vi "DC Dfficiency_noTorqueInput.vi"(0 "data":waveform(dbl)[](array[waveform])=[{"t0"=timestamp(3695322048.688499 s since 1904-01-01), "dt"=0.01, "Y"=[27.030278258476777, 27.030278258476777, 27.030278258476777, 27.030278258476777, 27.030278258476777, 27.030278258476777], "attributes"=variant("NI_ChannelName"=variant(string "T_comp_in"), "NI_UnitDescription"=variant(string "Deg C"))}, {"t0"=timestamp(3695322048.688499 s since 1904-01-01), "dt"=0.01, "Y"=[101.4755306317151, 101.4755306317151, 101.4755306317151, 101.4755306317151, 101.4755306317151, 101.4755306317151], "attributes"=variant("NI_ChannelName"=variant(string "T_comp_out"), "NI_UnitDescription"=variant(string "Deg C"))}, {"t0"=timestamp(3695322048.688499 s since 1904-01-01), "dt"=0.01, "Y"=[74.8524982036163, 74.8524982036163, 74.8524982036163, 74.8524982036163, 74.8524982036163, 74.8524982036163], "attributes"=variant("NI_ChannelName"=variant(string "T_int"), "NI_UnitDescription"=variant(string "Deg C"))}, {"t0"=timestamp(3695322048.688499 s since 1904-01-01), "dt"=0.01, "Y"=[49.22287356053607, 49.22287356053607, 49.22287356053607, 49.22287356053607, 49.22287356053607, 49.22287356053607], "attributes"=variant("NI_ChannelName"=variant(string "T_vapor"), "NI_UnitDescription"=variant(string "Deg C"))}, {"t0"=timestamp(3695322048.688499 s since 1904-01-01), "dt"=0.01, "Y"=[22.86482944196074, 22.86482944196074, 22.86482944196074, 22.86482944196074, 22.86482944196074, 22.86482944196074], "attributes"=variant("NI_ChannelName"=variant(string "T_cd_out"), "NI_UnitDescription"=variant(string "Deg C"))}, {"t0"=timestamp(3695322048.688499 s since 1904-01-01), "dt"=0.01, "Y"=[22.390101755165144, 22.390101755165144, 22.390101755165144, 22.390101755165144, 22.390101755165144, 22.390101755165144], "attributes"=variant("NI_ChannelName"=variant(string "T_liq"), "NI_UnitDescription"=variant(string "Deg C"))}, {"t0"=timestamp(3695322048.688499 s since 1904-01-01), "dt"=0.01, "Y"=[22.35929456927789, 22.35929456927789, 22.35929456927789, 22.35929456927789, 22.35929456927789, 22.35929456927789], "attributes"=variant("NI_ChannelName"=variant(string "T_cf_in"), "NI_UnitDescription"=variant(string "Deg C"))}, {"t0"=timestamp(3695322048.688499 s since 1904-01-01), "dt"=0.01, "Y"=[25.57925048739495, 25.57925048739495, 25.57925048739495, 25.57925048739495, 25.57925048739495, 25.57925048739495], "attributes"=variant("NI_ChannelName"=variant(string "T_cf_out"), "NI_UnitDescription"=variant(string "Deg C"))}, {"t0"=timestamp(3695322048.688499 s since 1904-01-01), "dt"=0.01, "Y"=[-56050.12537094423, -56050.12537094423, -56050.12537094423, -56050.12537094423, -56050.12537094423, -56050.12537094423], "attributes"=variant("NI_ChannelName"=variant(string "T_cj_in"), "NI_UnitDescription"=variant(string "Deg C"))}, {"t0"=timestamp(3695322048.688499 s since 1904-01-01), "dt"=0.01, "Y"=[-56050.12537094423, -56050.12537094423, -56050.12537094423, -56050.12537094423, -56050.12537094423, -56050.12537094423], "attributes"=variant("NI_ChannelName"=variant(string "T_cj_out"), "NI_UnitDescription"=variant(string "Deg C"))}, {"t0"=timestamp(3695322048.688499 s since 1904-01-01), "dt"=0.01, "Y"=[25.130324713777938, 25.130324713777938, 25.130324713777938, 25.130324713777938, 25.130324713777938, 25.130324713777938], "attributes"=variant("NI_ChannelName"=variant(string "T_amb"), "NI_UnitDescription"=variant(string "Deg C"))}, {"t0"=timestamp(3695322048.688499 s since 1904-01-01), "dt"=0.01, "Y"=[89.88480677591595, 89.88480677591595, 89.88480677591595, 89.88480677591595, 89.88480677591595, 89.88480677591595], "attributes"=variant("NI_ChannelName"=variant(string "T_os_out"), "NI_UnitDescription"=variant(string "Deg C"))}, {"t0"=timestamp(3695322048.688499 s since 1904-01-01), "dt"=0.01, "Y"=[66.71254591399129, 66.71254591399129, 66.71254591399129, 66.71254591399129, 66.71254591399129, 66.71254591399129], "attributes"=variant("NI_ChannelName"=variant(string "Housing Upstream"), "NI_UnitDescription"=variant(string "Deg C"))}, {"t0"=timestamp(3695322048.688499 s since 1904-01-01), "dt"=0.01, "Y"=[76.6589685879223, 76.6589685879223, 76.6589685879223, 76.6589685879223, 76.6589685879223, 76.6589685879223], "attributes"=variant("NI_ChannelName"=variant(string "Housing Middle"), "NI_UnitDescription"=variant(string "Deg C"))}, {"t0"=timestamp(3695322048.688499 s since 1904-01-01), "dt"=0.01, "Y"=[72.22038712366484, 72.22038712366484, 72.22038712366484, 72.22038712366484, 72.22038712366484, 72.22038712366484], "attributes"=variant("NI_ChannelName"=variant(string "Housing Downstream"), "NI_UnitDescription"=variant(string "Deg C"))}, {"t0"=timestamp(3695322048.688499 s since 1904-01-01), "dt"=0.01, "Y"=[-56050.12537094423, -56050.12537094423, -56050.12537094423, -56050.12537094423, -56050.12537094423, -56050.12537094423], "attributes"=variant("NI_ChannelName"=variant(string "NC3"), "NI_UnitDescription"=variant(string "Deg C"))}, {"t0"=timestamp(3695322048.688499 s since 1904-01-01), "dt"=0.01, "Y"=[0.003513029999999999, 0.002876085999999999, 0.002876085999999999, 0.0031945579999999993, 0.003513029999999999, 0.0031945579999999993], "attributes"=variant("NI_ChannelName"=variant(string "I_comp"))}, {"t0"=timestamp(3695322048.688499 s since 1904-01-01), "dt"=0.01, "Y"=[-0.7271732700000002, -0.48073149000000015, -0.7176947400000002, -0.42386031000000013, -0.4996885500000002, -0.3575106000000001], "attributes"=variant("NI_ChannelName"=variant(string "V_comp"))}, {"t0"=timestamp(3695322048.6884995 s since 1904-01-01), "dt"=0.01, "Y"=[144.98366426907117, 143.44548240534618, 150.02890078208918, 149.29057348750118, 147.44475525103118, 148.98293711475617], "attributes"=variant("NI_ChannelName"=variant(string "P_comp_suc"))}, {"t0"=timestamp(3695322048.688514 s since 1904-01-01), "dt"=0.01, "Y"=[540.496080804404, 544.7419326821, 550.28000034866, 519.3898895862919, 528.989206874996, 534.711876797108], "attributes"=variant("NI_ChannelName"=variant(string "P_comp_dis"))}, {"t0"=timestamp(3695322048.688529 s since 1904-01-01), "dt"=0.01, "Y"=[298.9543326272059, 297.3539518286699, 310.8340824009539, 287.9363263603619, 299.4467574882939, 300.67781964101385], "attributes"=variant("NI_ChannelName"=variant(string "P_comp_int"))}, {"t0"=timestamp(3695322048.6885443 s since 1904-01-01), "dt"=0.01, "Y"=[0.004162377994999999, 0.004139413934999999, 0.0041033275549999994, 0.004067241174999999, 0.0039868669649999995, 0.003972104355], "attributes"=variant("NI_ChannelName"=variant(string "m_dot_wf"))}, {"t0"=timestamp(3695322048.6884995 s since 1904-01-01), "dt"=0.01, "Y"=[-4.3651000000322516e-06, -0.0002668923000000322, 0.00037301774999996774, -5.358895000003224e-05, 2.845079999996776e-05, 0.0007339926499999677], "attributes"=variant("NI_ChannelName"=variant(string "m_dot_oil"))}, {"t0"=timestamp(3695322048.688559 s since 1904-01-01), "dt"=0.01, "Y"=[-517.556345519233, -517.089975251254, -515.7332617444059, -509.2040779927, -517.0475779541649, -516.8779887658089], "attributes"=variant("NI_ChannelName"=variant(string "P_housing"))}], 1 "S_v":dbl=0.0196978, 2 "Override (V)":dbl=205.0, 3 "Override Speed Entry?":i32=1, 4 "Mass Flow [kg/s]":i32=21, 5 "error in (no error)":errorcluster, 6 "Working Fluid":string="R245FA.FLD", 7 "Speed (RPM)":i32, 9 "Comp Pressure Out (PSI)":i32=19, 10 "?":path=path "C:/Users/ASITest/Desktop/REFPROP", 11 "Override Power Entry?":i32=1, 13 "Override (RPM)":dbl=3550.0, 14 "Comp Pressure In (PSI)":i32=18, 15 "Current":i32=16, 16 "Override (A)":dbl=3.3, 17 "Voltage":i32=17, 18 "Comp Temp In (C)":i32) -> (12 "Eff.":waveform(dbl)[](graph)=[{"t0"=timestamp(3695322048.658514 s since 1904-01-01), "dt"=0.01, "Y"=[0.4567975829903178]}, {"t0"=timestamp(3695322048.658514 s since 1904-01-01), "dt"=0.01, "Y"=[8.028990231944996e-05]}], 19 "error out":errorcluster)   [LabVIEW 2016]
uses:
  <vilib>/Utility/error.llb/DialogType.ctl
panel:
  out "Enthalpy_in":dbl=425.28689493486974
  out "Entropy_in":dbl=1.7599617768753537
  out "Density_in":dbl=8.45632520959761
  out "m_dot":dbl=0.003972104355
  out "N [rev/s]":dbl=59.166666666666664
  out "V_eff":dbl=0.4030362849415085
  out "Eff. 2":waveform(dbl)[](array[waveform])=[{"t0"=timestamp(3695322048.658514 s since 1904-01-01), "dt"=0.01, "Y"=[0.4567975829903178]}, {"t0"=timestamp(3695322048.658514 s since 1904-01-01), "dt"=0.01, "Y"=[8.028990231944996e-05]}]
  out "W_dot_shaft":dbl=1126.3978938578941
  out "Ideal Enthalpy":dbl=448.05527380609516
  out "delta_Enthalpy":dbl=22.768378871225423
  out "Isen_Eff":dbl=8.028990231944996e-05
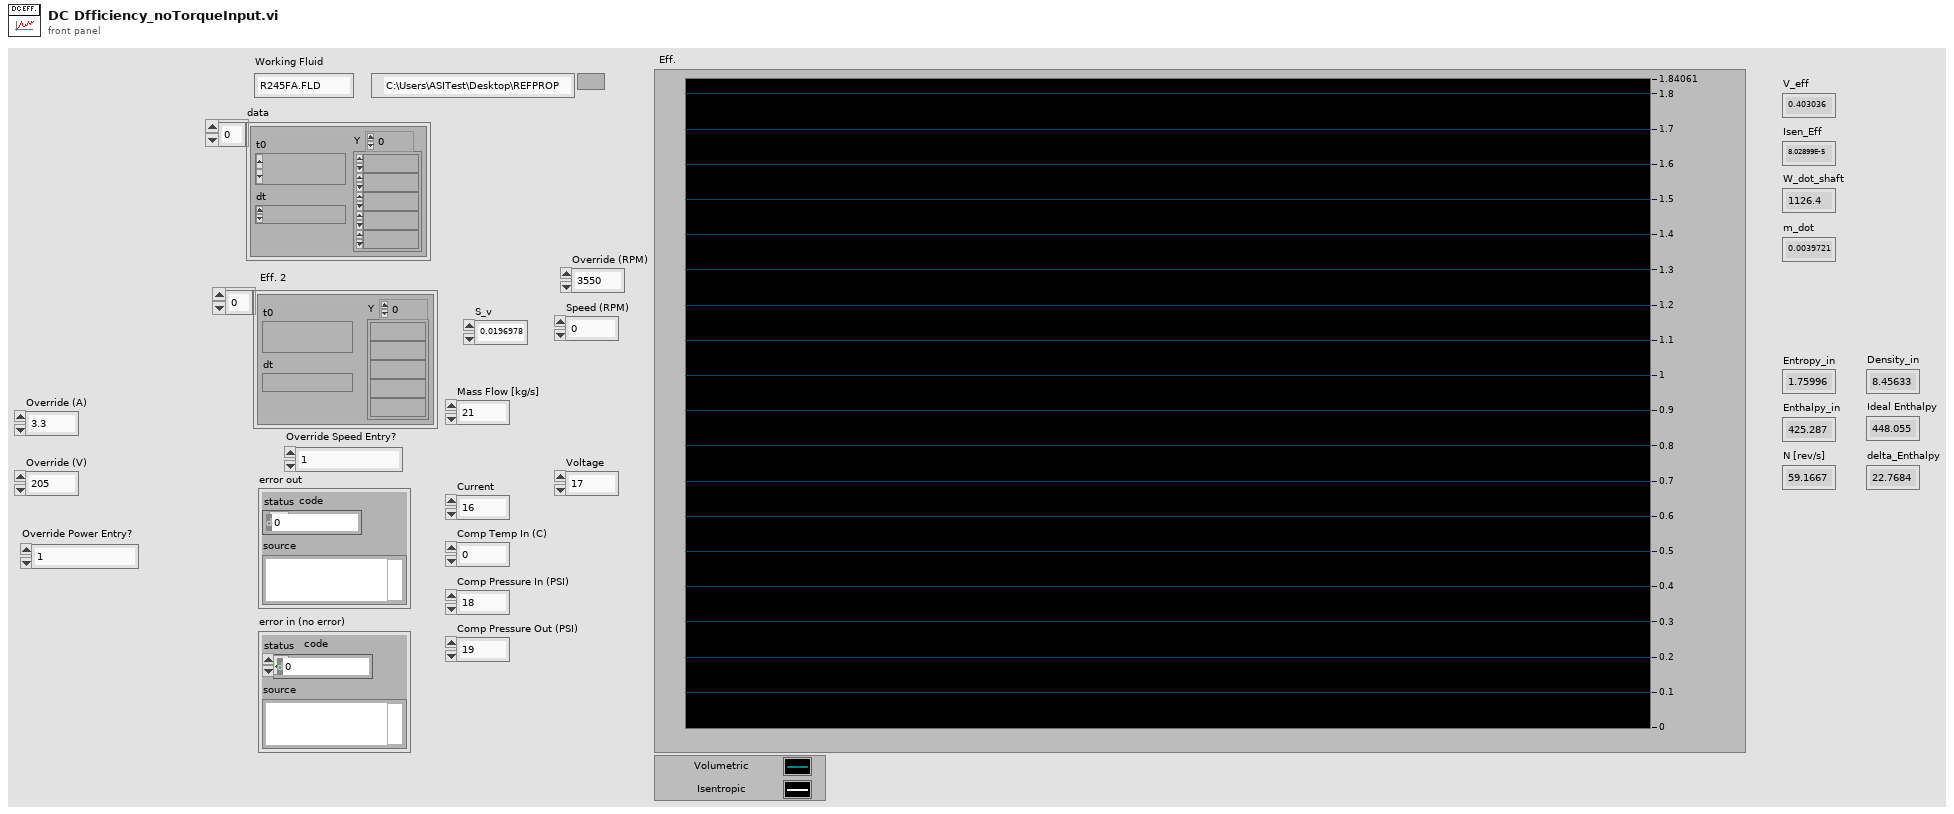
[diagram p1: front panel]
types:
  T1 = typedef "DialogType.ctl" = u16
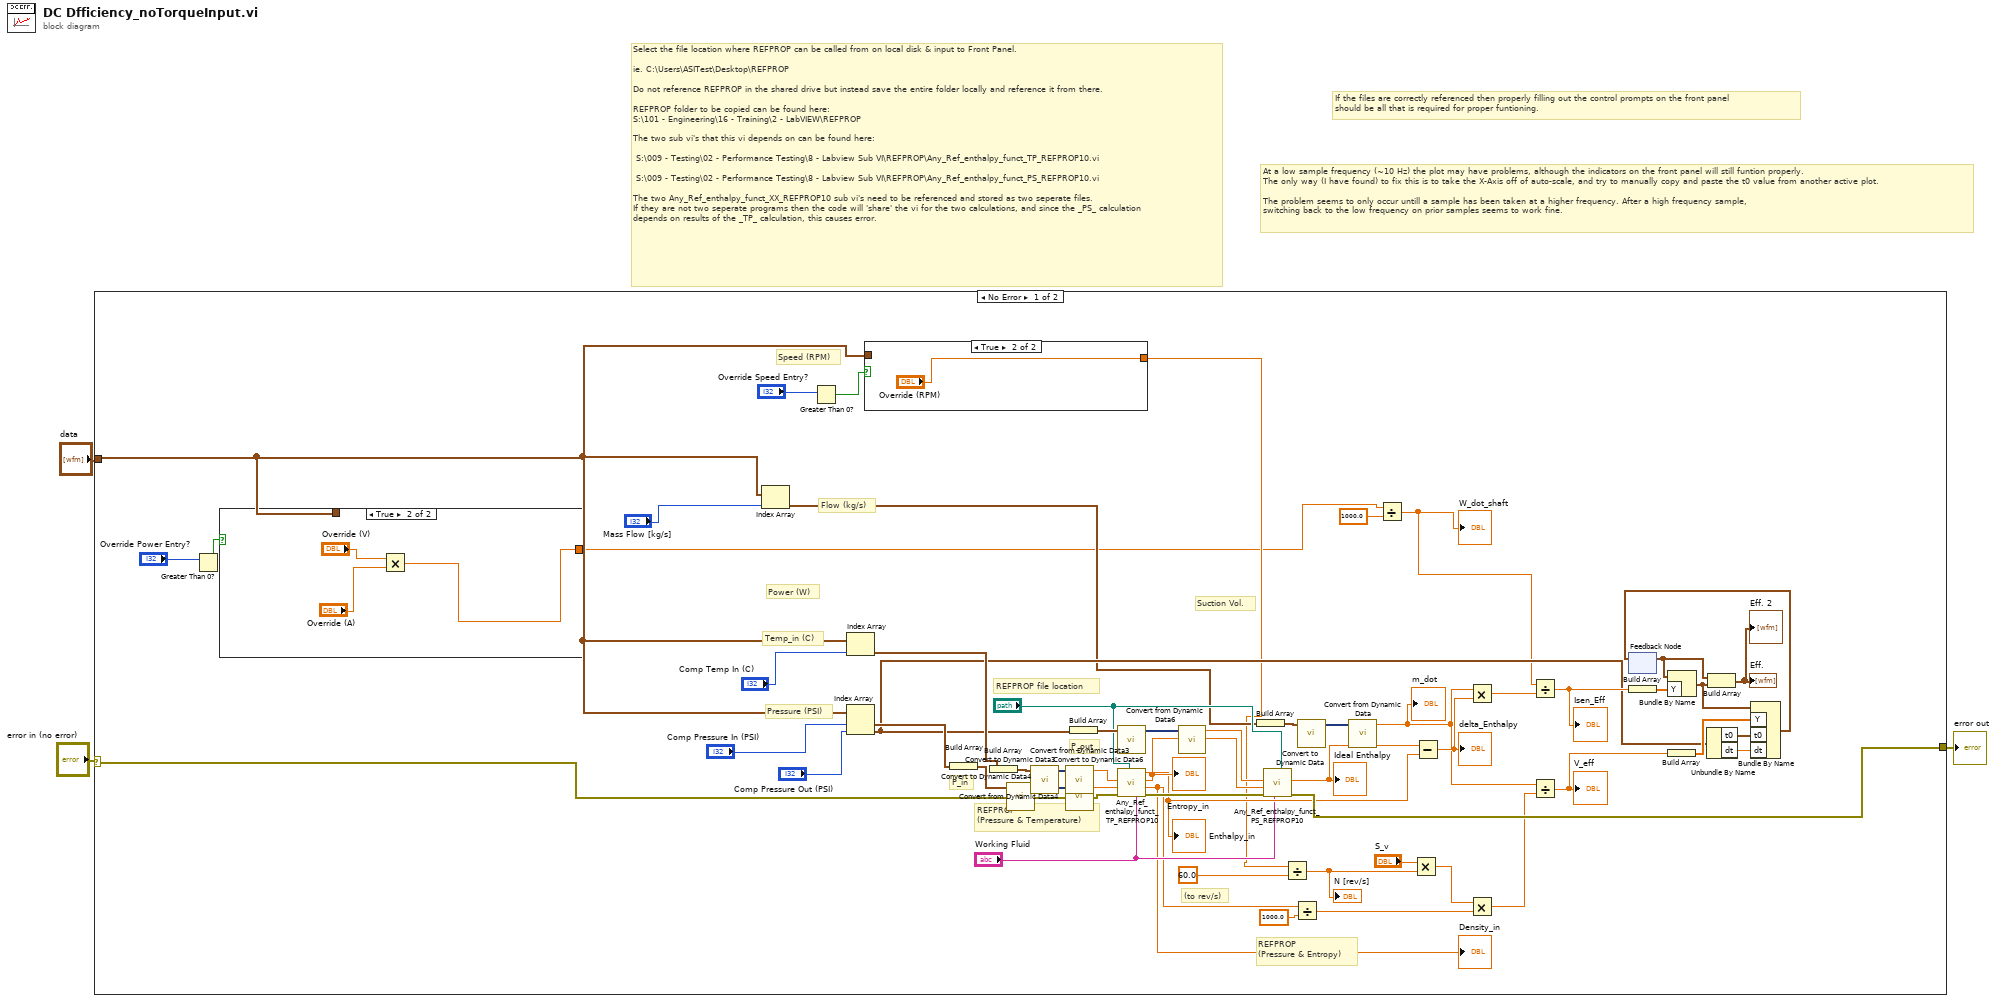
[diagram p0: block diagram]
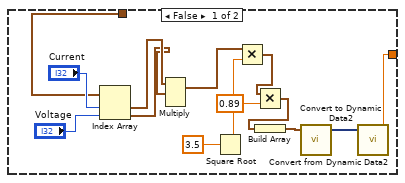
[diagram p2: hidden frame]
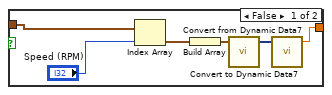
[diagram p3: hidden frame]
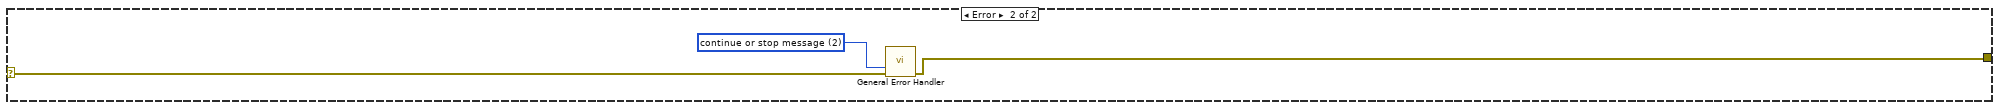
[diagram p4: hidden frame]
diagram:
  # "At a low sample frequency (~10 Hz) the plot may have problems, although the indicators on the front panel will still funtion properly.\nThe only way (I have found) to fix this is to take the X-Axis off of auto-scale, and try to manually copy and paste the t0 value from another active plot. \n\nThe problem seems to only occur untill a sample has been taken at a higher frequency. After a high frequency sample, \nswitching back to the low frequency on prior samples seems to work fine."
  # "If the files are correctly referenced then properly filling out the control prompts on the front panel \nshould be all that is required for proper funtioning."
  # "Select the file location where REFPROP can be called from on local disk & input to Front Panel.\n\nie. C:\\Users\\ASITest\\Desktop\\REFPROP\n\nDo not reference REFPROP in the shared drive but instead save the entire folder locally and reference it from there.\n\nREFPROP folder to be copied can be found here: \nS:\\101 - Engineering\\16 - Training\\2 - LabVIEW\\REFPROP\n\nThe two sub vi's that this vi depends on can be found here:\n\n S:\\009 - Testing\\02 - Performance Testing\\8 - Labview Sub VI\\REFPROP\\Any_Ref_enthalpy_funct_TP_REFPROP10.vi\n\n S:\\009 - Testing\\02 - Performance Testing\\8 - Labview Sub VI\\REFPROP\\Any_Ref_enthalpy_funct_PS_REFPROP10.vi\n\nThe two Any_Ref_enthalpy_funct_XX_REFPROP10 sub vi's need to be referenced and stored as two seperate files. \nIf they are not two seperate programs then the code will 'share' the vi for the two calculations, and since the _PS_ calculation\ndepends on results of the _TP_ calculation, this causes error."
  n1 = case shown="No Error" "error in (no error)" {
    selector: "error in (no error)" -> [w47 w85]
    tunnel: "data" -> [w9 _]
    tunnel: [w44 w86] -> w1
    frame No Error {
      # "Suction Vol."
      # "(to rev/s)"
      # "REFPROP\n(Pressure & Temperature)"
      # "REFPROP\n(Pressure & Entropy)"
      # "REFPROP file location"
      # "P_in"
      # "P_out"
      # "Power (W)"
      # "Pressure (PSI)"
      # "Temp_in (C)"
      # "Speed (RPM)"
      # "Flow (kg/s)"
      n2 = Greater Than 0?(x="Override Power Entry?") -> (x > 0?=w8:bool)
      n3 = case shown="True" w8 {
        tunnel: [w61 w75] -> w6
        tunnel: w9 -> [w72 _]
        frame False {
          n4 = Index Array(array=w72, index #1="Current", index #2="Voltage") -> (element #1=w68:waveform(dbl), element #2=w67:waveform(dbl))
          n5 = Multiply(1:w67, 2:w68) -> (0:w71:waveform(dbl))  [unwired: 1 in, 1 out]
          n6 = Square Root(x=3.5) -> (sqrt(x)=w70:dbl)
          n7 = Multiply(x=w71, y=w70) -> (x*y=w65:waveform(dbl))
          n8 = Multiply(x=w65, y=0.89) -> (x*y=w62:waveform(dbl))
          n9 = Build Array(w62) -> (w63:waveform(dbl)[])
          n10 = call "Convert to Dynamic Data2"("Array of Waveforms"=w63) -> ("Dynamic Data Type"=w64:dynamicdata)  [unwired: 3 in]
          n11 = call "Convert from Dynamic Data2"("Dynamic Data Type"=w64) -> ("Scalar"=w61:dbl)  [unwired: 3 in]
        }
        frame True {
          n12 = Multiply(x="Override (V)", y="Override (A)") -> (x*y=w75:dbl)
        }
      }
      n13 = Index Array(array=w9, index="Mass Flow [kg/s]") -> (element=w22:waveform(dbl))
      n14 = Greater Than 0?(x="Override Speed Entry?") -> (x > 0?=w24:bool)
      n15 = Index Array(array=w9, index="Comp Temp In (C)") -> (element=w53:waveform(dbl))
      n16 = Index Array(array=w9, index #1="Comp Pressure In (PSI)", index #2="Comp Pressure Out (PSI)") -> (element #1=w51:waveform(dbl), element #2=w29:waveform(dbl))
      n17 = case shown="True" w24 {
        tunnel: [w78 "Override (RPM)"] -> w16
        tunnel: w9 -> [w80 _]
        frame False {
          n18 = Index Array(array=w80, index="Speed (RPM)") -> (element=w82:waveform(dbl))
          n19 = Build Array(w82) -> (w83:waveform(dbl)[])
          n20 = call "Convert to Dynamic Data7"("Array of Waveforms"=w83) -> ("Dynamic Data Type"=w79:dynamicdata)  [unwired: 3 in]
          n21 = call "Convert from Dynamic Data7"("Dynamic Data Type"=w79, "Channel"=w79) -> ("Scalar"=w78:dbl)  [unwired: 2 in]
        }
        frame True {
        }
      }
      n22 = Build Array(w51) -> (w54:waveform(dbl)[])
      n23 = Build Array(w53) -> (w57:waveform(dbl)[])
      n24 = call "Convert to Dynamic Data4"("Array of Waveforms"=w54) -> ("Dynamic Data Type"=w55:dynamicdata)  [unwired: 3 in]
      n25 = call "Convert to Dynamic Data3"("Array of Waveforms"=w57) -> ("Dynamic Data Type"=w58:dynamicdata)  [unwired: 3 in]
      n26 = call "Convert from Dynamic Data3"("Dynamic Data Type"=w58) -> ("Scalar"=w56:dbl)  [unwired: 3 in]
      n27 = call "Convert from Dynamic Data4"("Dynamic Data Type"=w55) -> ("Scalar"=w19:dbl)  [unwired: 3 in]
      n28 = Build Array(w29) -> (w49:waveform(dbl)[])
      n29 = call "Convert to Dynamic Data6"("Array of Waveforms"=w49) -> ("Dynamic Data Type"=w50:dynamicdata)  [unwired: 3 in]
      n30 = call "Any_Ref_enthalpy_funct_TP_REFPROP10.vi"("Input Temperature [C]"=w56, "Input Pressure [kPa]"=w19, "error in (no error)"=w47, 4:"?", "Fluidofinterest"="Working Fluid") -> ("Enthalpy [kJ/kg]"=w39:dbl, "Entropy"=w46:dbl, "Density"=w13:dbl, "error out"=w45:errorcluster)  [unwired: 2 in]
      "Enthalpy_in" <- w39
      "Entropy_in" <- w46
      "Density_in" <- w13
      n31 = call "Convert from Dynamic Data6"("Dynamic Data Type"=w50) -> ("Scalar"=w18:dbl)  [unwired: 3 in]
      n32 = Build Array(w22) -> (w20:waveform(dbl)[])
      n33 = call "Any_Ref_enthalpy_funct_PS_REFPROP10.vi"("Pressure Out (kPa)"=w18, "S_in"=w46, "error in (no error)"=w45, "Fluidofinterest"="Working Fluid", 5:"?") -> ("h2_s"=w40:dbl, "error out"=w44:errorcluster)  [unwired: 4 in]
      "Ideal Enthalpy" <- w40
      n34 = Divide(x=w16, y=60.0) -> (x/y=w15:dbl)
      "N [rev/s]" <- w15
      n35 = Divide(x=w13, y=1000.0) -> (x/y=w11:dbl)
      n36 = call "Convert to Dynamic Data"("Array of Waveforms"=w20) -> ("Dynamic Data Type"=w21:dynamicdata)  [unwired: 3 in]
      n37 = call "Convert from Dynamic Data"("Dynamic Data Type"=w21) -> ("Scalar"=w14:dbl)  [unwired: 3 in]
      "m_dot" <- w14
      n38 = Divide(x=w6, y=1000.0) -> (x/y=w5:dbl)
      "W_dot_shaft" <- w5
      n39 = Multiply(x="S_v", y=w15) -> (x*y=w59:dbl)
      n40 = Subtract(x=w40, y=w39) -> (x-y=w43:dbl)
      "delta_Enthalpy" <- w43
      n41 = Multiply(x=w14, y=w43) -> (x*y=w4:dbl)
      n42 = Multiply(x=w59, y=w11) -> (x*y=w17:dbl)
      n43 = Divide(x=w5, y=w4) -> (x/y=w42:dbl)
      "Isen_Eff" <- w42
      n44 = Divide(x=w14, y=w17) -> (x/y=w52:dbl)
      "V_eff" <- w52
      n45 = feedback #1() -> (w26:waveform(dbl))  [unwired: 1 in]
      n46 = Build Array(w42) -> (w41:dbl[])
      n47 = Bundle By Name ("Build Waveform")(cluster=w26, "Y"=w41) -> (w28:waveform(dbl))
      n48 = Build Array(w52) -> (w33:dbl[])
      n49 = Unbundle By Name(w29) -> ("t0"=w34:timestamp, "dt"=w35:dbl)
      n50 = Build Array(w26, w28) -> (→"Eff. 2" →"Eff.":waveform(dbl)[])
      n51 = Bundle By Name ("Build Waveform")(cluster=w28, "Y"=w33, "t0"=w34, "dt"=w35) -> (w27:waveform(dbl))
      n52 = feedback-in #1(w27) -> ()
    }
    frame Error {
      w87 = T1 2 items=["no dialog", "OK message", "continue or stop message", "OK message + warnings", "continue/stop + warnings"] ("type of dialog (OK msg:1)")
      n53 = call <vilib>:"General Error Handler.vi"("type of dialog (OK msg:1)"=w87, "error in (no error)"=w85) -> ("error out"=w86:errorcluster)  [unwired: 9 in, 4 out]
    }
  }
  "error out" <- w1
